vi "TSPopup.Initialize.vi"(8 "error in (no error)":errorcluster, 9 "Font Size":u32, 10 "Popup Cluster Ref":refnum<vi>, 11 "TSPopup in":refnum<class "TSPopup.lvclass">) -> (0 "error out":errorcluster, 2 "Popup Event":refnum<user-event>, 3 "TSPopup out":refnum<class "TSPopup.lvclass">)   [LabVIEW 2016, in "TSPopup.lvlib" / "TSPopup.lvclass"]
doc: "Initializes the Type Sensitive Popup. Needs to be run at the beginning of the program.\n\n<B>Popup Cluster Ref</B> - Reference to the Popup Cluster which needs to be placed on the Front Panel of the VI. (cluster can be placed anywhere, but must be frontmost)\n<B>Font Size</B> - Sets the font size of popups with text.\n\n<B>Popup Event</B> - User Event reference. This must be registered by an Event Structure. It will fire when the popup data entry is complete.\n\nType Sensitive Popup \nCopyright © 2007, J. David Saunders\nAll rights reserved."
uses:
  <userlib>/TSPopup/TSPopup.lvclass
  <userlib>/TSPopup/Private/TSPopup.Popup Results.ctl
  <userlib>/TSPopup/Private/TSPopup.Monitor Register Data.ctl
  <userlib>/TSPopup/Private/TSPopup.Event Enum.ctl
  <userlib>/TSPopup/TSPopup.Popup Call Parameters.ctl
  <userlib>/TSPopup/TSPopup.Data Type.ctl
  <userlib>/TSPopup/TSPopup.lvclass/TSPopup.ctl
  <userlib>/TSPopup/Private/TSPopup.Monitor Events.vi
panel:
  # "Type Sensitive Popup \nCopyright © 2007, J. David Saunders\nAll rights reserved."
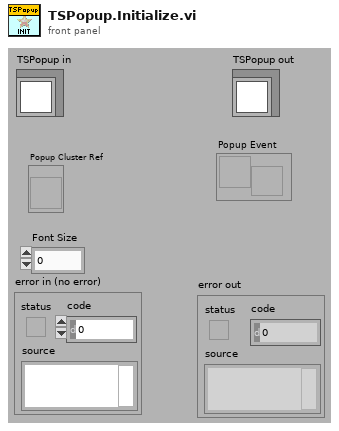
[diagram p1: front panel]
types:
  T1 = typedef "TSPopup.lvlib/TSPopup.lvclass/TSPopup.Popup Call Parameters.ctl" = cluster{"Prop Type":T2, "Initial Value":variant, "Caption Strings":string[], "Ring Strings":string[], "Cell Rect":cluster{"left":i16, "top":i16, "right":i16, "bottom":i16}, "Mouse Coords":cluster{"x":i16, "y":i16}, "Call Data":variant}
  T2 = typedef "TSPopup.lvlib/TSPopup.lvclass/TSPopup.Data Type.ctl" = enum16{"Unkown", "NO POPUP", "String", "Integer", "Float", "Color", "Boolean", "Ring", "Captioned String", "Captioned Integer", "Button Color", "2 Int Cluster", "4 Int Cluster", "check"}
  T3 = typedef "TSPopup.lvlib/TSPopup.lvclass/TSPopup.Monitor Register Data.ctl" = cluster{"Control":refnum<vi>, "Events":T4[]}
  T4 = typedef "TSPopup.lvlib/TSPopup.lvclass/TSPopup.Event Enum.ctl" = enum16{"Nothing", "Enter Key Accept", "Escape Key Cancel", "Mouse Outside Accept", "Mouse Outside Cancel", "Mouse Move Accept", "Mouse Move Cancel", "Mouse Leave Cancel", "Value Change Accept", "Lose Focus Cancel", "Cancel Button", "Accept Button"}
  T5 = typedef "TSPopup.lvlib/TSPopup.lvclass/TSPopup.Popup Results.ctl" = cluster{"Valid?":bool, "Value Changed?":bool, "Popup Value":variant, "Call Data":variant}
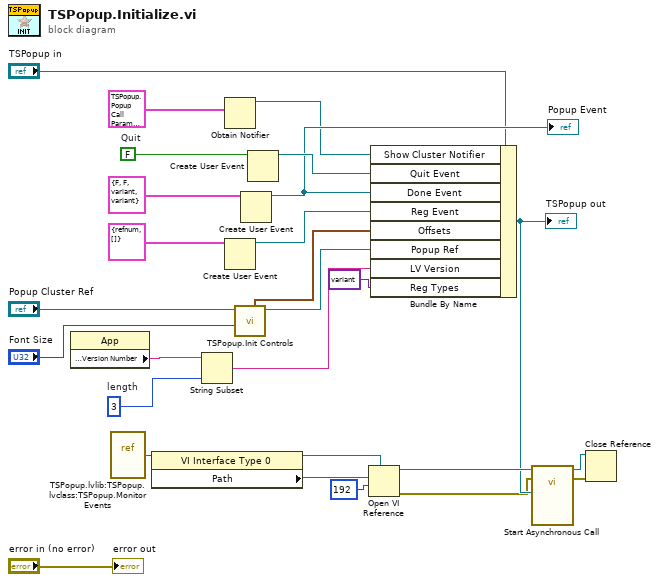
[diagram p0: block diagram]
diagram:
  w15 = 3  # length
  w18 = FALSE  # Quit
  n1 = property class="App"() -> ("Application:Version Number"=w16:string)  [unwired: 2 in, 2 out]
  n2 = vi-ref "TSPopup.lvlib:TSPopup.lvclass:TSPopup.Monitor Events.vi"() -> (w8:refnum<vi>)
  n3 = property class="VI Interface Type 0"(reference=w8) -> (reference out=w5:refnum<vi>, "Path"=w7:path)  [unwired: 1 in, 1 out]
  n4 = String Subset(string=w16, length (rest)=w15) -> (substring=w21:string)  [unwired: 1 in]
  n5 = Obtain Notifier(notification data type=T1 {"Prop Type"=enum."Unkown", "Initial Value"=variant, "Caption Strings"=[], "Ring Strings"=[], "Cell Rect"={"left"=0, "top"=0, "right"=0, "bottom"=0}, "Mouse Coords"={"x"=0, "y"=0}, "Call Data"=variant} ("Show Cluster")) -> (notifier out=w10:refnum<notifier>)  [unwired: 3 in, 2 out]
  n6 = Create User Event(user event datatype=T3 {"Control"=refnum, "Events"=[]} ("Reg. Data (type only)")) -> (user event=w24:refnum<user-event>)  [unwired: 1 in, 1 out]
  n7 = call <userlib>:"TSPopup.Init Controls.vi"("Font Size"="Font Size", "Popup Cluster Ref"="Popup Cluster Ref") -> ("dup ref"=w22:refnum<vi>, "Offsets"=w23:cluster{"Left":i32, "Top":i32}[])  [unwired: 8 in]
  n8 = Create User Event(user event datatype=T5 {"Valid?"=FALSE, "Value Changed?"=FALSE, "Popup Value"=variant, "Call Data"=variant} ("Popup Results (type only)")) -> (user event=w14:refnum<user-event>)  [unwired: 1 in, 1 out]
  "Popup Event" <- w14
  n9 = Create User Event(user event datatype=w18) -> (user event=w25:refnum<user-event>)  [unwired: 1 in, 1 out]
  n10 = Open VI Reference(type specifier VI Refnum (for type only)=w5, vi path=w7, options=192) -> (vi reference=w9:refnum<vi>, error out=w2:errorcluster)  [unwired: 3 in]
  n11 = Bundle By Name(cluster="TSPopup in", "Show Cluster Notifier"=w10, "Quit Event"=w25, "Done Event"=w14, "Reg Event"=w24, "Offsets"=w23, "Popup Ref"=w22, "LV Version"=w21, "Reg Types"=variant ("Variant")) -> (w4:refnum<class "TSPopup.lvclass">)
  "TSPopup out" <- w4
  n12 = call-by-ref "Start Asynchronous Call"(reference=w9, error in=w2, "TSPopup"=w4) -> (reference out=w3:refnum<vi>, error out=w1:errorcluster)  [unwired: 11 in]
  n13 = Close Reference(reference=w3, error in (no error)=w1) -> ()  [unwired: 1 out]
  "error out" <- "error in (no error)"
